vi "Get T.vi"(8 "error in (no error)":errorcluster, 11 "Thermometer in":refnum<class "Thermometer.lvclass">) -> (0 "error out":errorcluster, 2 "T":dbl, 3 "Thermometer out":refnum<class "Thermometer.lvclass">)   [LabVIEW 2016, in "Hardware.lvlib" / "Thermometer.lvlib" / "Thermometer.lvclass"]
uses:
  <userlib>/Common Components/Hardware/Thermometer/Thermometer.lvclass
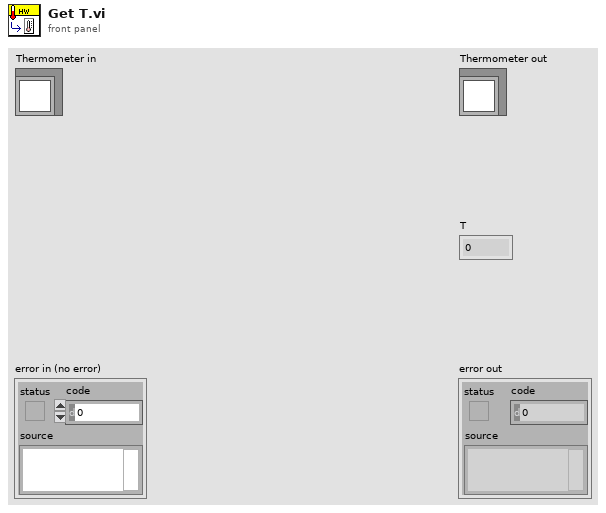
[diagram p1: front panel]
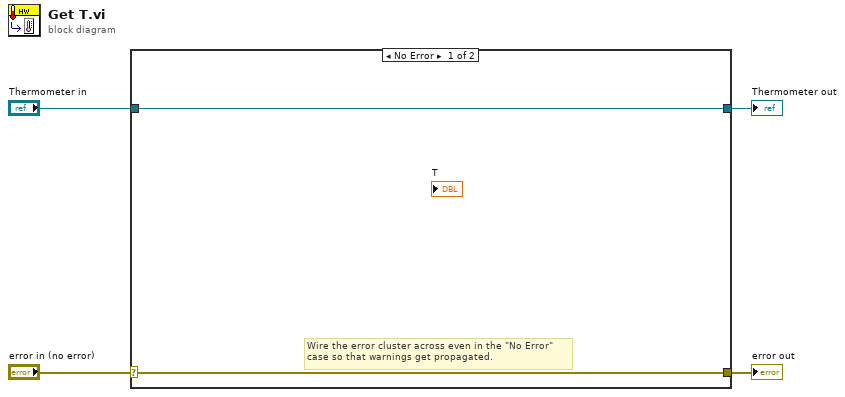
[diagram p0: block diagram]
diagram:
  n1 = case shown="No Error" "error in (no error)" {
    selector: "error in (no error)" -> [w5 w8]
    tunnel: [w5 w8] -> w3
    tunnel: [w6 w7] -> w1
    tunnel: "Thermometer in" -> [w6 w7]
    frame No Error {
      # "Wire the error cluster across even in the \"No Error\"\ncase so that warnings get propagated."
    }
    frame Error {
    }
  }
  "error out" <- w3
  "Thermometer out" <- w1
